vi "CTRE_CANTalonSRX_Open.vi"(6 "Invert":bool, 7 "Control Period (ms)":u8=10, 8 "error in":errorcluster, 9 "Master Device Number":u8, 10 "Device Number":u8, 11 "Control Mode":T1) -> (0 "error out":errorcluster, 3 "CAN Talon SRX Ref":T2={"DeviceStatus"={"status"=FALSE, "code"=0, "source"=""}, "Type"=enum."PWM", "PWM"={"PWM Channel"=enum."PWM 1", "DeadBand"={"Name"="", "maxPositivePwm"=0, "minPositivePwm"=0, "centerPwm"=0, "maxNegativePwm"=0, "minNegativePwm"=0, "angularRange"=0}}, "CAN"={"Device Number"=0, "SetOutput VI Ref"=variant(enum8{"Percent VBus", "Current", "Speed", "Position", "Voltage"} enum."Percent VBus"), "GetOutput VI Ref"=variant(refnum<k1> refnum), "Enable VI Ref"=variant(dbl 12.0), "Disable VI Ref"=variant(enum8{"Percent VBus", "Speed", "Position", "Slave", "Unchanged / Invalid", "Voltage Compensation", "Current", "Motion Profile"} enum."Percent VBus"), "Data"=variant}, "Invert"=FALSE})   [LabVIEW 2016]
doc: "Creates a reference to the CAN-connected Talon SRX motor controller you specify. You must open a reference before using any other VIs on this palette. After you open a reference to the Talon SRX motor controller, you can use the other Talon SRX VIs to configure and control the Talon SRX. This reference is compatible with the WPI Robotics Motor VIs.\n\n<B>Control Mode</B> is the desired control mode of the Talon SRX.\n\n<B>Device Number</B> is the Talon SRX Device ID on the CAN bus.\n\n<B>Master Device Number</B> is the CAN bus Device ID of the master controller that this controller is to follow.\n\n<B>Invert</B> enables/disables inverting the motor when using the WPI Robotics SetOutput.vi."
uses:
  <vilib>/Rock Robotics/WPI/MotorControl/WPI_MotorControlDeviceRef.ctl
  <vilib>/Rock Robotics/WPI/MotorControl/WPI_MotorControlType.ctl
  <vilib>/Rock Robotics/SystemInterfaces/DIO/FPGA_DIOPWMChannel.ctl
  <vilib>/Rock Robotics/WPI/PWM/WPI_PWMDeadband.ctl
  <vilib>/Rock Robotics/WPI/ThirdParty/CanMotor/CTRLib-LV-TalonSRX/CTRE_CANTalonSRX_ControlMode.ctl
  <vilib>/Rock Robotics/WPI/ThirdParty/CanMotor/CTRLib-LV-TalonSRX/TalonSRXDevRefData.ctl
  <vilib>/Rock Robotics/WPI/ThirdParty/CanMotor/CTRLib-LV-TalonSRX/CTRE_CANTalonSRX_UsageTypes.ctl
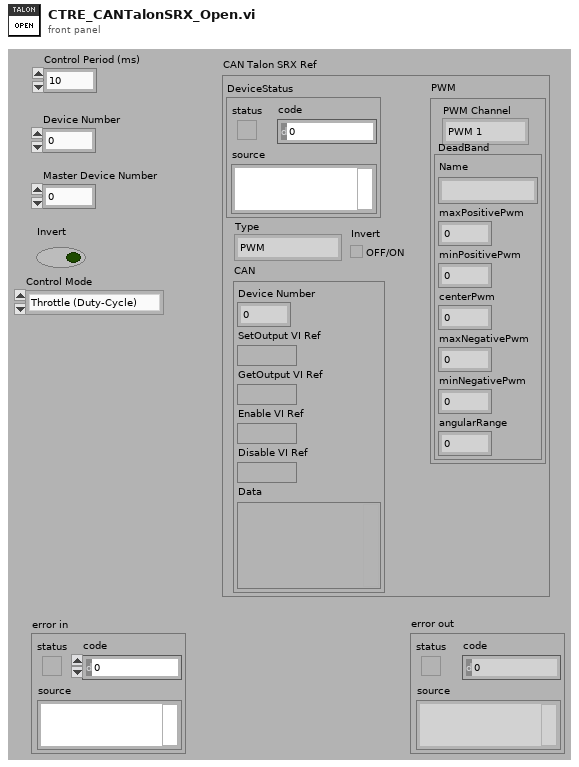
[diagram p1: front panel]
types:
  T1 = typedef "CTRE_CANTalonSRX_ControlMode.ctl" = enum16{"Throttle (Duty-Cycle)", "Position Closed-Loop", "Velocity Closed-Loop", "Current Closed-Loop", "Voltage Compensation", "Slave Follower", "Motion Profile", "Motion Magic"}
  T2 = typedef "WPI_MotorControlDeviceRef.ctl" = cluster{"DeviceStatus":errorcluster, "Type":T3, "PWM":cluster{"PWM Channel":T4, "DeadBand":T5}, "CAN":cluster{"Device Number":u8, "SetOutput VI Ref":variant, "GetOutput VI Ref":variant, "Enable VI Ref":variant, "Disable VI Ref":variant, "Data":variant}, "Invert":bool}
  T3 = typedef "WPI_MotorControlType.ctl" = enum16{"PWM", "CAN"}
  T4 = typedef "FPGA_DIOPWMChannel.ctl" = enum8{"PWM 0", "PWM 1", "PWM 2", "PWM 3", "PWM 4", "PWM 5", "PWM 6", "PWM 7", "PWM 8", "PWM 9", "PWM MXP 0", "PWM MXP 1", "PWM MXP 2", "PWM MXP 3", "PWM MXP 4", "PWM MXP 5", "PWM MXP 6", "PWM MXP 7", "PWM MXP 8", "PWM MXP 9", "Invalid"}
  T5 = typedef "WPI_PWMDeadband.ctl" = cluster{"Name":string, "maxPositivePwm":i32, "minPositivePwm":i32, "centerPwm":i32, "maxNegativePwm":i32, "minNegativePwm":i32, "angularRange":u16}
  T6 = typedef "TalonSRXDevRefData.ctl" = cluster{"Library":path, "handle":u64, "Talon SRX Mode":T1, "UsageFrame":u32, "RefNumName":string}
  T7 = typedef "CTRE_CANTalonSRX_UsageTypes.ctl" = u32
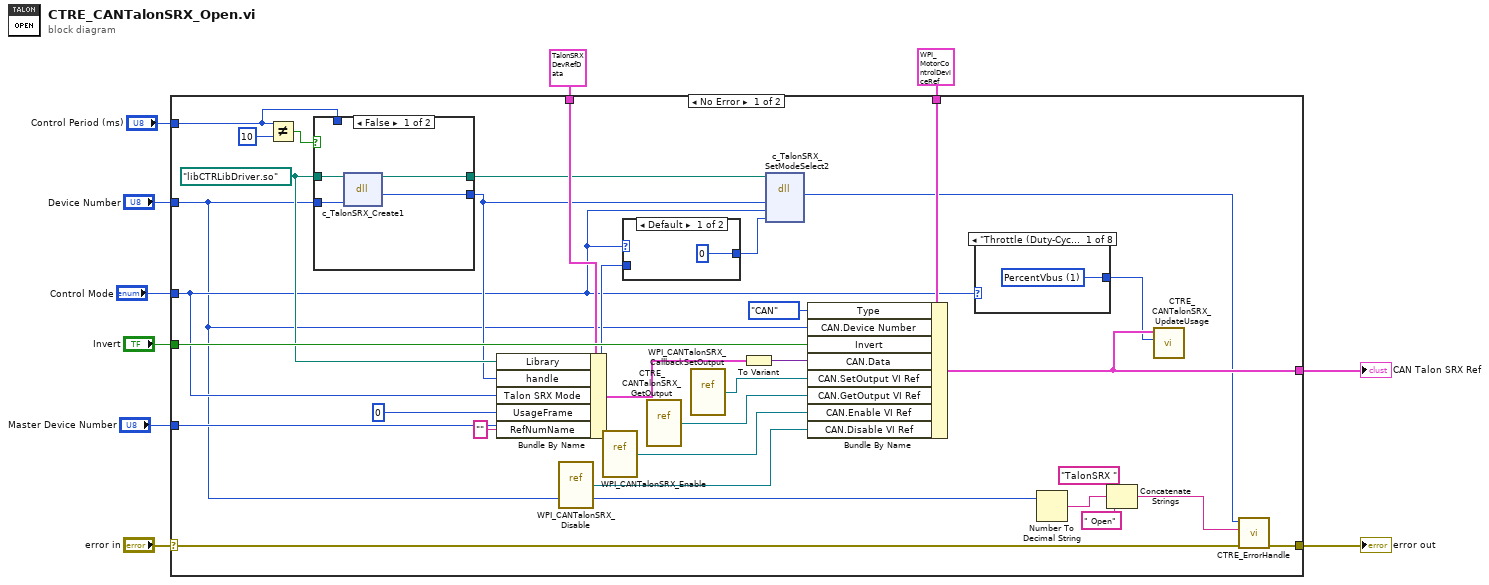
[diagram p0: block diagram]
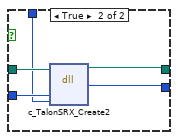
[diagram p2: hidden frame]
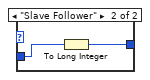
[diagram p3: hidden frame]
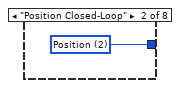
[diagram p4: hidden frame]
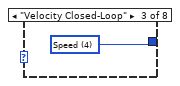
[diagram p5: hidden frame]
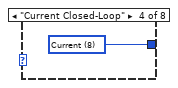
[diagram p6: hidden frame]
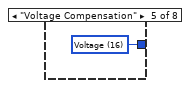
[diagram p7: hidden frame]
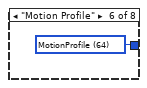
[diagram p8: hidden frame]
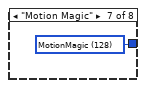
[diagram p9: hidden frame]
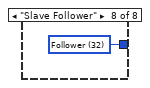
[diagram p10: hidden frame]
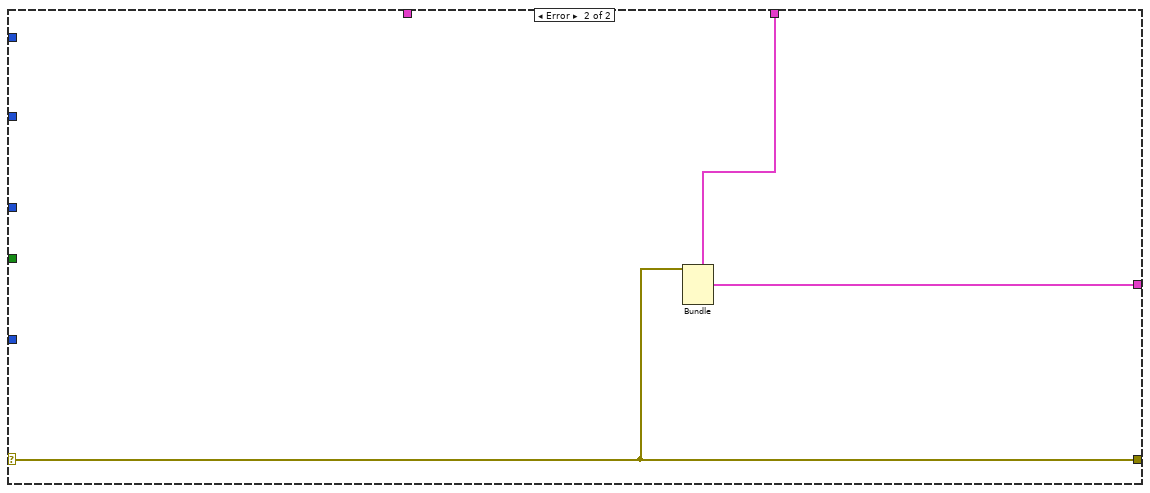
[diagram p11: hidden frame]
diagram:
  n1 = case shown="No Error" "error in" {
    selector: "error in" -> [w24 w62]
    tunnel: [w23 w62] -> w10
    tunnel: "Invert" -> [w38 _]
    tunnel: T2 {"DeviceStatus"={"status"=FALSE, "code"=0, "source"=""}, "Type"=enum."CAN", "PWM"={"PWM Channel"=enum."PWM 1", "DeadBand"={"Name"="", "maxPositivePwm"=0, "minPositivePwm"=0, "centerPwm"=0, "maxNegativePwm"=0, "minNegativePwm"=0, "angularRange"=0}}, "CAN"={"Device Number"=0, "SetOutput VI Ref"=variant(refnum<vi> refnum), "GetOutput VI Ref"=variant(refnum<vi> refnum), "Enable VI Ref"=variant(refnum<vi> refnum), "Disable VI Ref"=variant(refnum<vi> refnum), "Data"=variant(cluster{"Control Mode":enum8{"Percent VBus", "Speed", "Position", "Slave", "Unchanged / Invalid", "Voltage Compensation", "Current", "Motion Profile"}, "Encoder Initial Position":dbl, "MaxVout":dbl} {"Control Mode"=enum."Percent VBus", "Encoder Initial Position"=0.0, "MaxVout"=12.0})}, "Invert"=FALSE} ("CAN Talon SRX Ref") -> [w41 w64]
    tunnel: "Device Number" -> [w13 _]
    tunnel: "Control Mode" -> [w21 _]
    tunnel: "Master Device Number" -> [w26 _]
    tunnel: [w34 w63] -> w2
    tunnel: T6 {"Library"=path "", "handle"=0, "Talon SRX Mode"=enum."Throttle (Duty-Cycle)", "UsageFrame"=0, "RefNumName"=""} -> [w29 _]
    tunnel: "Control Period (ms)" -> [w18 _]
    frame No Error {
      w32 = path "libCTRLibDriver.so" ("path in")
      n2 = Not Equal?(x=w18, y=u8 10) -> (x != y?=w19:bool)
      n3 = case shown="False" w19 {
        tunnel: w13 -> [w45 w49]
        tunnel: w32 -> [w44 w50]
        tunnel: [w43 w46] -> w28
        tunnel: [w42 w47] -> w27
        tunnel: w18 -> [_ w48]
        frame False {
          n4 = dll-call lib="?" fn="c_TalonSRX_Create1"(path in=w44, "deviceNumber"=w45) -> (path out=w42:path, "return type"=w43:u64)  [unwired: 3 in, 1 out]
        }
        frame True {
          n5 = dll-call lib="?" fn="c_TalonSRX_Create2"(path in=w50, "deviceNumber"=w49, "controlPeriodMs"=w48) -> (path out=w47:path, "return type"=w46:u64)  [unwired: 4 in, 1 out]
        }
      }
      n6 = Bundle By Name(cluster=w29, "Library"=w32, "handle"=w28, "Talon SRX Mode"=w21, "UsageFrame"=u32 0, "RefNumName"="") -> (w30:T6)
      n7 = vi-ref <vilib>:"WPI_CANTalonSRX_Disable.vi"() -> (w35:refnum<vi>)
      n8 = vi-ref <vilib>:"WPI_CANTalonSRX_Enable.vi"() -> (w36:refnum<vi>)
      n9 = case shown="Default" w21 {
        tunnel: w26 -> [_ w53]
        tunnel: [0 w52] -> w25
        frame Default {
        }
        frame "Slave Follower" {
          n10 = To Long Integer(number=w53) -> (32bit integer=w52:i32)
        }
      }
      n11 = vi-ref <vilib>:"CTRE_CANTalonSRX_GetOutput.vi"() -> (w37:refnum<vi>)
      n12 = vi-ref <vilib>:"WPI_CANTalonSRX_CallbackSetOutput.vi"() -> (w39:refnum<vi>)
      n13 = To Variant(anything=w30) -> (Variant=w31:variant)
      n14 = dll-call lib="?" fn="c_TalonSRX_SetModeSelect2"(path in=w27, "handle"=w28, "modeSelect"=w21, "demand"=w25) -> ("return type"=w17:i32)  [unwired: 5 in, 2 out]
      n15 = Bundle By Name(cluster=w41, "Type"=WPI_MotorControlType."CAN", "CAN.Device Number"=w13, "Invert"=w38, "CAN.Data"=w31, "CAN.SetOutput VI Ref"=w39, "CAN.GetOutput VI Ref"=w37, "CAN.Enable VI Ref"=w36, "CAN.Disable VI Ref"=w35) -> (w34:T2)
      n16 = case shown="\"Throttle (Duty-Cycle)\", Default" w21 {
        tunnel: [w54 w55 w56 w57 w58 w59 w60 w61] -> w33
        frame "Throttle (Duty-Cycle)", Default {
          w54 = T7 1 items=["Default"=0, "PercentVbus"=1, "Position"=2, "Speed"=4, "Current"=8, "Voltage"=16, "Follower"=32, "MotionProfile"=64, "MotionMagic"=128, "VRampRate"=4194304, "CurrentLimit"=8388608, "ZeroSensorI"=16777216, "ZeroSensorF"=33554432, "ZeroSensorR"=67108864, "ForwardLimitSwitch"=134217728, "ReverseLimitSwitch"=268435456, "ForwardSoftLimit"=536870912, "ReverseSoftLimit"=1073741824, "MultiProfile"=2147483648]
        }
        frame "Position Closed-Loop" {
          w55 = T7 2 items=["Default"=0, "PercentVbus"=1, "Position"=2, "Speed"=4, "Current"=8, "Voltage"=16, "Follower"=32, "MotionProfile"=64, "MotionMagic"=128, "VRampRate"=4194304, "CurrentLimit"=8388608, "ZeroSensorI"=16777216, "ZeroSensorF"=33554432, "ZeroSensorR"=67108864, "ForwardLimitSwitch"=134217728, "ReverseLimitSwitch"=268435456, "ForwardSoftLimit"=536870912, "ReverseSoftLimit"=1073741824, "MultiProfile"=2147483648]
        }
        frame "Velocity Closed-Loop" {
          w56 = T7 4 items=["Default"=0, "PercentVbus"=1, "Position"=2, "Speed"=4, "Current"=8, "Voltage"=16, "Follower"=32, "MotionProfile"=64, "MotionMagic"=128, "VRampRate"=4194304, "CurrentLimit"=8388608, "ZeroSensorI"=16777216, "ZeroSensorF"=33554432, "ZeroSensorR"=67108864, "ForwardLimitSwitch"=134217728, "ReverseLimitSwitch"=268435456, "ForwardSoftLimit"=536870912, "ReverseSoftLimit"=1073741824, "MultiProfile"=2147483648]
        }
        frame "Current Closed-Loop" {
          w57 = T7 8 items=["Default"=0, "PercentVbus"=1, "Position"=2, "Speed"=4, "Current"=8, "Voltage"=16, "Follower"=32, "MotionProfile"=64, "MotionMagic"=128, "VRampRate"=4194304, "CurrentLimit"=8388608, "ZeroSensorI"=16777216, "ZeroSensorF"=33554432, "ZeroSensorR"=67108864, "ForwardLimitSwitch"=134217728, "ReverseLimitSwitch"=268435456, "ForwardSoftLimit"=536870912, "ReverseSoftLimit"=1073741824, "MultiProfile"=2147483648]
        }
        frame "Voltage Compensation" {
          w58 = T7 16 items=["Default"=0, "PercentVbus"=1, "Position"=2, "Speed"=4, "Current"=8, "Voltage"=16, "Follower"=32, "MotionProfile"=64, "MotionMagic"=128, "VRampRate"=4194304, "CurrentLimit"=8388608, "ZeroSensorI"=16777216, "ZeroSensorF"=33554432, "ZeroSensorR"=67108864, "ForwardLimitSwitch"=134217728, "ReverseLimitSwitch"=268435456, "ForwardSoftLimit"=536870912, "ReverseSoftLimit"=1073741824, "MultiProfile"=2147483648]
        }
        frame "Motion Profile" {
          w59 = T7 64 items=["Default"=0, "PercentVbus"=1, "Position"=2, "Speed"=4, "Current"=8, "Voltage"=16, "Follower"=32, "MotionProfile"=64, "MotionMagic"=128, "VRampRate"=4194304, "CurrentLimit"=8388608, "ZeroSensorI"=16777216, "ZeroSensorF"=33554432, "ZeroSensorR"=67108864, "ForwardLimitSwitch"=134217728, "ReverseLimitSwitch"=268435456, "ForwardSoftLimit"=536870912, "ReverseSoftLimit"=1073741824, "MultiProfile"=2147483648]
        }
        frame "Motion Magic" {
          w60 = T7 128 items=["Default"=0, "PercentVbus"=1, "Position"=2, "Speed"=4, "Current"=8, "Voltage"=16, "Follower"=32, "MotionProfile"=64, "MotionMagic"=128, "VRampRate"=4194304, "CurrentLimit"=8388608, "ZeroSensorI"=16777216, "ZeroSensorF"=33554432, "ZeroSensorR"=67108864, "ForwardLimitSwitch"=134217728, "ReverseLimitSwitch"=268435456, "ForwardSoftLimit"=536870912, "ReverseSoftLimit"=1073741824, "MultiProfile"=2147483648]
        }
        frame "Slave Follower" {
          w61 = T7 32 items=["Default"=0, "PercentVbus"=1, "Position"=2, "Speed"=4, "Current"=8, "Voltage"=16, "Follower"=32, "MotionProfile"=64, "MotionMagic"=128, "VRampRate"=4194304, "CurrentLimit"=8388608, "ZeroSensorI"=16777216, "ZeroSensorF"=33554432, "ZeroSensorR"=67108864, "ForwardLimitSwitch"=134217728, "ReverseLimitSwitch"=268435456, "ForwardSoftLimit"=536870912, "ReverseSoftLimit"=1073741824, "MultiProfile"=2147483648]
        }
      }
      n17 = Number To Decimal String(number=w13) -> (decimal integer string=w15:string)  [unwired: 1 in]
      n18 = Concatenate Strings("TalonSRX " ("string"), w15, " Open" ("string")) -> (w12:string)
      n19 = call <vilib>:"CTRE_CANTalonSRX_UpdateUsage.vi"("Usage"=w33, "CAN Talon SRX Ref"=w34) -> ()  [unwired: 9 in, 1 out]
      n20 = call <vilib>:"CTRE_ErrorHandle.vi"("error in"=w24, "origin"=w12, "code"=w17) -> ("error out"=w23:errorcluster)  [unwired: 8 in]
    }
    frame Error {
      n21 = Bundle(cluster=w64, "DeviceStatus"=w62) -> (w63:T2)  [unwired: 4 in]
    }
  }
  "CAN Talon SRX Ref" <- w2
  "error out" <- w10
